vi "__SP_mk_peak.vi"(4 "GIPB番号":string="18") -> (0 "pow out":dbl format="%.4f", 1 "Freq out":dbl format="%.4f")   [LabVIEW 2017]
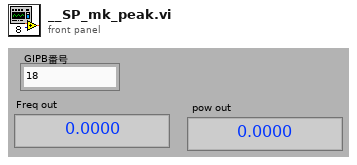
[diagram p1: front panel]
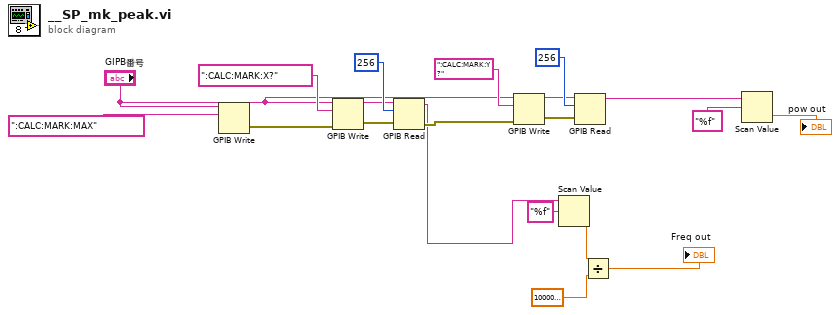
[diagram p0: block diagram]
diagram:
  n1 = GPIB Write(0:"GIPB番号", 1:":CALC:MARK:MAX") -> (6:w16:errorcluster)  [unwired: 3 in, 1 out]
  n2 = GPIB Write(0:"GIPB番号", 1:":CALC:MARK:X?", 3:w16) -> (6:w14:errorcluster)  [unwired: 2 in, 1 out]
  n3 = GPIB Read(0:"GIPB番号", 1:256, 3:w14) -> (5:w6:string, 7:w10:errorcluster)  [unwired: 2 in, 1 out]
  n4 = GPIB Write(0:"GIPB番号", 1:":CALC:MARK:Y?", 3:w10) -> (6:w11:errorcluster)  [unwired: 2 in, 1 out]
  n5 = Scan Value(string=w6, format string="%f" ("形式文字列")) -> (value=w5:dbl)  [unwired: 1 in, 1 out]
  n6 = GPIB Read(0:"GIPB番号", 1:256, 3:w11) -> (5:w2:string)  [unwired: 2 in, 2 out]
  n7 = Divide(x=w5, y=1000000000.0) -> (x/y=→"Freq out":dbl)
  n8 = Scan Value(string=w2, format string="%f" ("形式文字列")) -> (value=→"pow out":dbl)  [unwired: 1 in, 1 out]
